vi "注册.vi"(8 "error in (no error)":errorcluster caption="错误输入（无错误）", 10 "数据值引用":refnum<data-value>, 11 "数据采集 输入":refnum<class "数据采集.lvclass"> caption="DNL_LabVIEW Object in") -> (0 "error out":errorcluster caption="错误输出", 3 "数据采集 输出":refnum<class "数据采集.lvclass"> caption="DNL_LabVIEW Object out")   [LabVIEW 2013, in "数据采集.lvclass"]
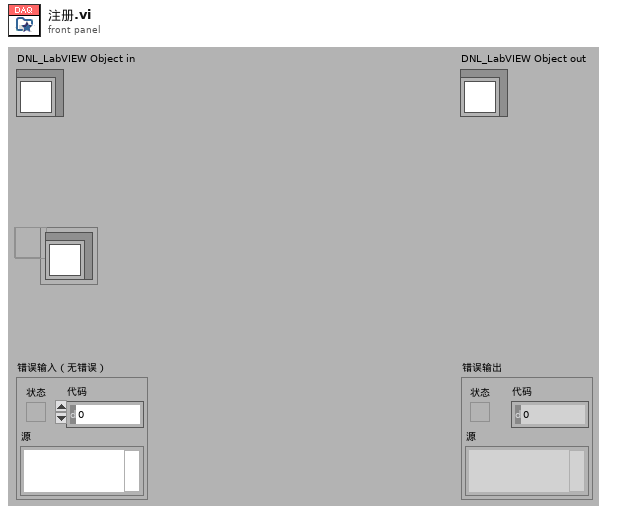
[diagram p1: front panel]
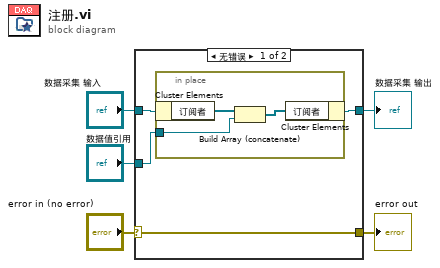
[diagram p0: block diagram]
diagram:
  n1 = case shown="无错误" "error in (no error)" {
    selector: "error in (no error)" -> [w6 w14]
    tunnel: [w6 w14] -> w4
    tunnel: "数据采集 输入" -> [w9 w13]
    tunnel: [w7 w13] -> w2
    tunnel: "数据值引用" -> [w8 _]
    frame No Error {
      n2 = in-place {
        in-place-border: w8 -> [w10]
        n3 = in-place-cluster #1(w9) -> ("订阅者"=w12:refnum<data-value>[])
        n4 = Build Array (concatenate)(w12, w10) -> (w11:refnum<data-value>[])
        n5 = in-place-cluster #1("订阅者"=w11) -> (w7:refnum<class "数据采集.lvclass">)
      }
    }
    frame Error {
    }
  }
  "error out" <- w4
  "数据采集 输出" <- w2
